vi "FPGA init.vi"(8 "error in":errorcluster) -> (0 "error out":errorcluster, 3 "FPGA VI Reference Out":refnum<k20>)   [LabVIEW 2019]
uses:
  <vilib>/FPGAPlugInAG/myRIO-1900/niLvFpga_Open_myRIO-1900.vi
  <vilib>/rvi/interface/common/dynamic/niFpgaDynamicAddResources.vi
  FPGA varible.vi
  <vilib>/rvi/interface/nirviOpenFPGA/nirviOpenFPGA.xnode
  3tires/FPGA Bitfiles/3tires_FPGATarget_FPGA-test001_3c7C1qXkvac.lvbitx
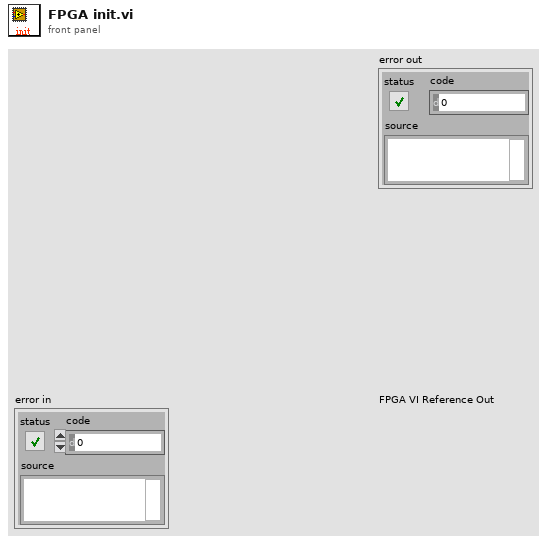
[diagram p1: front panel]
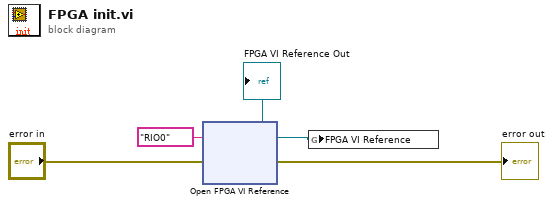
[diagram p0: block diagram]
diagram:
  n1 = xnode "Open FPGA VI Reference"("error in"="error in", "resource name"=tag "RIO0") -> ("FPGA VI Reference Out"=w2:refnum<k20>, "error out"=→"error out":errorcluster)
  "FPGA VI Reference Out" <- w2
  n2 = global write "FPGA varible.vi" "FPGA VI Reference"(w2) -> ()
